vi "MMEM_CAT.vi"(0 "VISA IN":refnum<visa-resource-name>, 1 "Folder":string, 5 "error in":errorcluster, 7 "Types":string(combo)) -> (14 "VISA Out":refnum<visa-resource-name>, 16 "Data":string, 19 "error out":errorcluster)   [LabVIEW 2018, in "PNA-X.lvlib"]
doc: "MMEMory:CATalog[:<char>]? [<folder>] \n1608\n\n(Read-only) Returns a comma-separated string of file names that are in the specified folder. If there \nare no files of the specified type, \"NO CATALOG\" is returned. Learn about File Types \nParameters \n<char> The type of files to list. Choose from: \nSTATe - Instrument states (.sta) \nCORRection - Calibration Data (.cal) \nCSARchive - Instrument state and calibration data (.csa) \nCSTate - Instrument state and link to Calibration data (.cst) \nIf unspecified then ALL file types (even unknown types) are listed. \n<folder> String - Any existing folder name. See Specifying Path Names \nExamples MMEM:CAT? 'lists all files from the current folder \nmmemory:catalog:correction? 'C:\\Program Files\\Agilent\\Network \nAnalyzer\\Documents' 'lists .cal files from the specified folder \nDefault Not applicable"
uses:
  PNA-X.lvlib
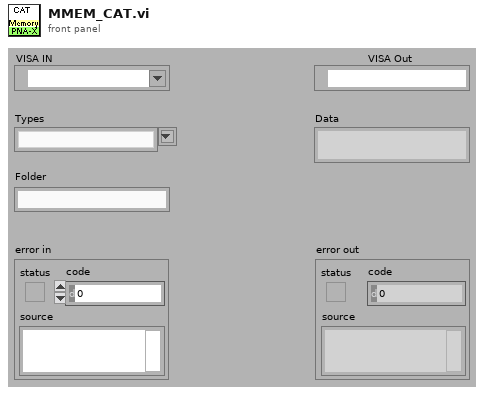
[diagram p1: front panel]
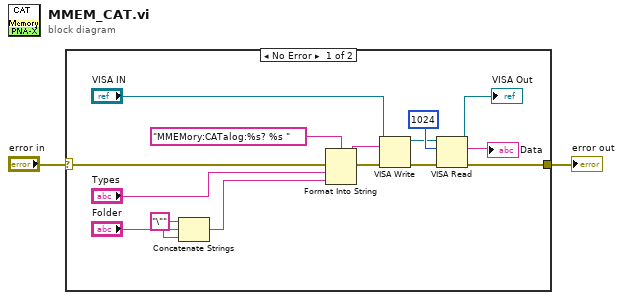
[diagram p0: block diagram]
diagram:
  n1 = case shown="No Error" "error in" {
    selector: "error in" -> [w17 w18]
    tunnel: [w9 w18] -> w1
    frame No Error {
      w3 = "\"" ("string")
      n2 = Concatenate Strings(w3, "Folder", w3) -> (w4:string)
      n3 = Format Into String(format string="MMEMory:CATalog:%s? %s " ("Cmdline"), error in=w17, "Types", w4) -> (resulting string=w15:string, error out=w16:errorcluster)  [unwired: 1 in]
      n4 = VISA Write(VISA resource name="VISA IN", write buffer=w15, error in (no error)=w16) -> (VISA resource name out=w10:refnum<visa-resource-name>, error out=w12:errorcluster)  [unwired: 1 out]
      n5 = VISA Read(VISA resource name=w10, byte count=1024, error in (no error)=w12) -> (VISA resource name out=→"VISA Out":refnum<visa-resource-name>, read buffer=→"Data":string, error out=w9:errorcluster)  [unwired: 1 out]
    }
    frame Error {
    }
  }
  "error out" <- w1
